vi "MotionProfiles_Start.vi"(8 "error in (no error)":errorcluster, 11 "MotionProfiles in":refnum<class "MotionProfiles.lvclass">) -> (0 "error out":errorcluster, 3 "MotionProfiles out":refnum<class "MotionProfiles.lvclass">)   [LabVIEW 2016, in "MotionProfiles.lvclass"]
uses:
  MotionProfiles.lvclass
  MotionProfiles.lvclass/MotionProfiles.ctl
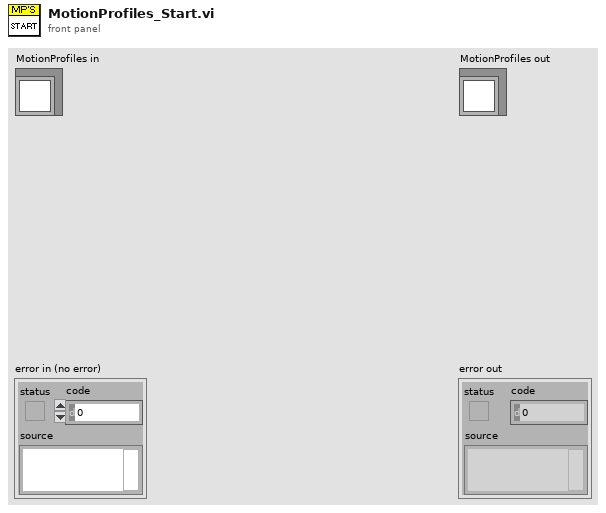
[diagram p1: front panel]
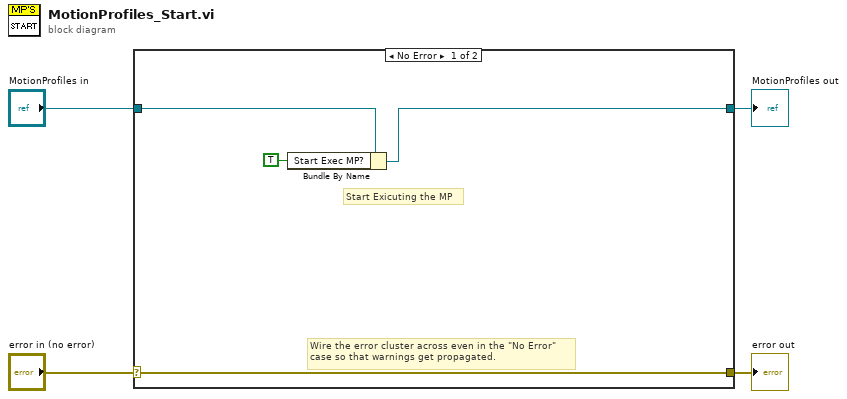
[diagram p0: block diagram]
diagram:
  n1 = case shown="No Error" "error in (no error)" {
    selector: "error in (no error)" -> [w8 w10]
    tunnel: [w8 w10] -> w3
    tunnel: [w5 w9] -> w1
    tunnel: "MotionProfiles in" -> [w7 w9]
    frame No Error {
      # "Start Exicuting the MP"
      # "Wire the error cluster across even in the \"No Error\"\ncase so that warnings get propagated."
      n2 = Bundle By Name(cluster=w7, "Start Exec MP?"=TRUE) -> (w5:refnum<class "MotionProfiles.lvclass">)
    }
    frame Error {
    }
  }
  "error out" <- w3
  "MotionProfiles out" <- w1
